vi "SetStringGetLength.vi"(10 "String":string) -> (2 "StringLength":i32)   [LabVIEW 2015]
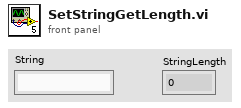
[diagram p1: front panel]
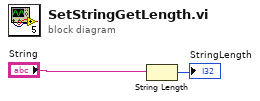
[diagram p0: block diagram]
diagram:
  n1 = String Length(string="String") -> (length=→"StringLength":i32)
